vi "FillControllerCombo.vi"(8 "error in (no error)":errorcluster, 10 "Device Array":T1(array[cluster]), 11 "Selected Controller:":refnum<vi>) -> (0 "error out":errorcluster)   [LabVIEW 2019]
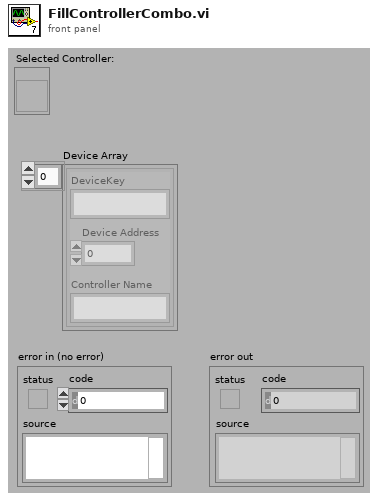
[diagram p1: front panel]
types:
  T1 = cluster{"DeviceKey":string, "Device Address":i32, "Controller Name":string}[]
  T2 = cluster{"DeviceKey":string, "Device Address":i32, "Controller Name":string}
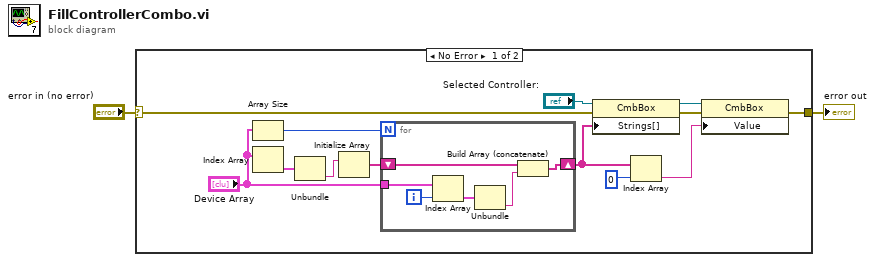
[diagram p0: block diagram]
diagram:
  n1 = case shown="No Error" "error in (no error)" {
    selector: "error in (no error)" -> [w3 w22]
    tunnel: [w4 w22] -> w1
    frame No Error {
      n2 = Array Size(array="Device Array") -> (size(s)=w10:i32)
      n3 = Index Array(array="Device Array") -> (element=w9:T2)  [unwired: 1 in]
      n4 = Unbundle(w9) -> ("Controller Name"=w7:string)  [unwired: 2 out]
      n5 = Initialize Array(w7) -> (w6:string[])  [unwired: 1 in]
      n6 = for {
        N: w10 -> [_]
        tunnel: "Device Array" -> [w21]
        shift-right: [w17] -> w5
        shift-left: w6 -> [w18]
        i -> [w20]
        n7 = Index Array(array=w21, index=w20) -> (element=w19:T2)
        n8 = Unbundle(w19) -> ("Controller Name"=w16:string)  [unwired: 2 out]
        n9 = Build Array (concatenate)(w18, w16) -> (w17:string[])
      }
      n10 = property class="CmbBox"(reference="Selected Controller:", error in=w3, "Strings[]"=w5) -> (reference out=w11:refnum<vi>, error out=w12:errorcluster)
      n11 = Index Array(array=w5, index=0) -> (element=w15:string)
      n12 = property class="CmbBox"(reference=w11, error in=w12, "Value"=w15) -> (error out=w4:errorcluster)  [unwired: 1 out]
    }
    frame Error {
    }
  }
  "error out" <- w1
